vi "Evaluate headers only from data files.vi"() -> ()   [LabVIEW 2017]
panel:
  out "String":string
  in  "stop":bool
  out "text":string
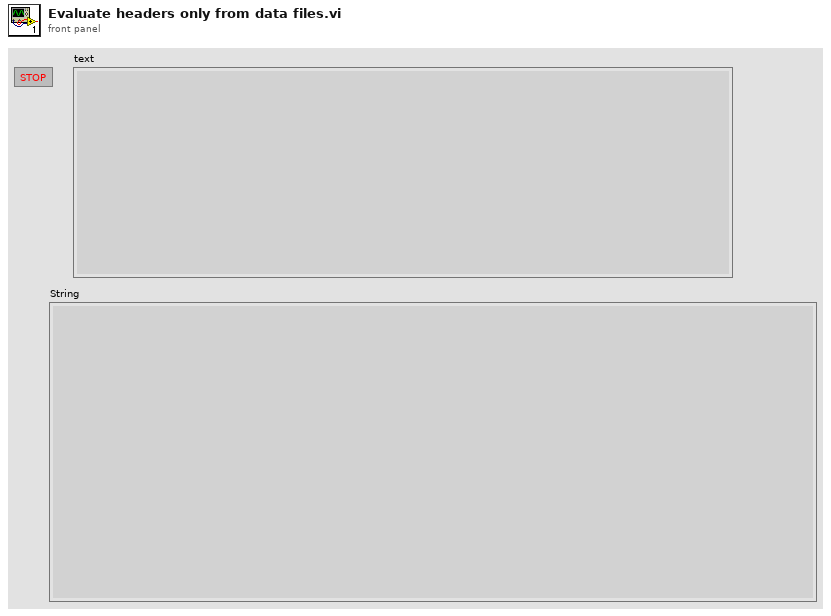
[diagram p1: front panel]
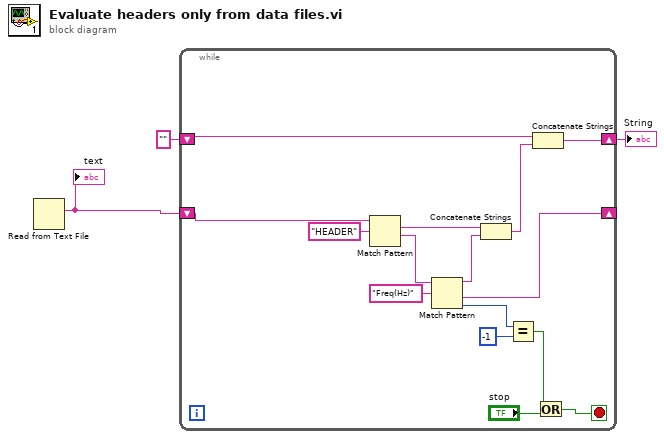
[diagram p0: block diagram]
diagram:
  n1 = Read from Text File() -> (text=w3:string)  [unwired: 4 in, 3 out]
  "text" <- w3
  n2 = while {
    shift-right: [w10] -> w1
    shift-left: "" -> [w9]
    shift-right: [w8] -> _
    shift-left: w3 -> [w17]
    stop <- w4 stop-if-true
    n3 = Match Pattern(string=w17, regular expression="HEADER") -> (match substring=w13:string, after substring=w14:string)  [unwired: 1 in, 2 out]
    n4 = Match Pattern(string=w14, regular expression="Freq(Hz)") -> (before substring=w12:string, after substring=w8:string, offset past match=w7:i32)  [unwired: 1 in, 1 out]
    n5 = Concatenate Strings(w13, w12) -> (w11:string)
    n6 = Equal?(x=w7, y=-1) -> (x = y?=w5:bool)
    n7 = Concatenate Strings(w9, w11) -> (w10:string)
    n8 = Or(x=w5, y="stop") -> (x .or. y?=w4:bool)
  }
  "String" <- w1
